vi "OCT Bscan Test_2.vi"() -> ()   [LabVIEW 2017]
panel:
  out "Intensity Graph":dbl[][](graph)
  in  "Data Range":T1={"Z start (pxl)"=1, "Z length (pxl)"=400}
  in  "# Cscan":i32
  in  "Save Path":path=path "E:/Jiarui/0212test"
  out "error out":errorcluster
  in  "Objective":u16(ring)=1 items=["5X LKM05", "10X LKM10", "20X LKM20", "10X LSM02"]
  in  "ROI Parameters":T2={"ROI (mm)"={"X (mm)"=1.0, "Y (mm)"=1.0}, "Shift (mm)"={"Xshift (mm)"=0.0, "Yshift (mm)"=0.0}}
  in  "Scan Parameters":T3={"# Scan"={"#Ascan"=400, "#Bscan"=400}, "# Rpt"={"#ARpt"=1, "#BRpt"=1}, "Aline Rate"=2, "# Extra"={"# ARpt_extra"=5, "#Brtn_extra"=80}} {"Aline Rate" items=["76 KHz", "146 KHz", "76 KHz", "28 KHz", "10 KHz"]}
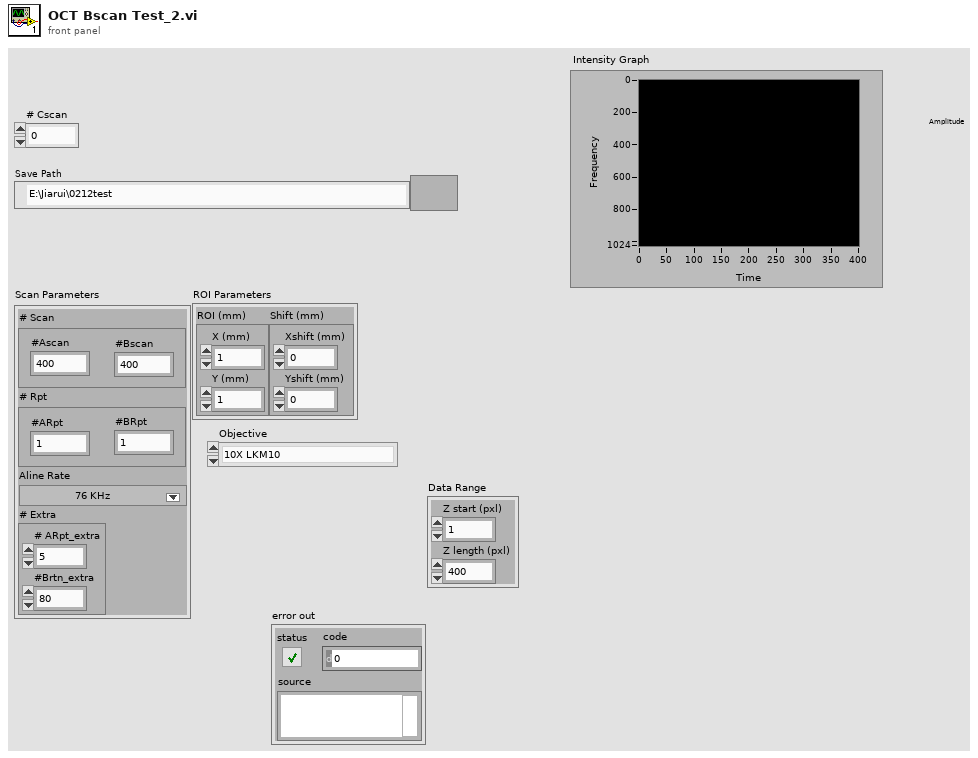
[diagram p1: front panel]
types:
  T1 = cluster{"Z start (pxl)":i32, "Z length (pxl)":i32}
  T2 = cluster{"ROI (mm)":cluster{"X (mm)":sgl, "Y (mm)":sgl}, "Shift (mm)":cluster{"Xshift (mm)":sgl, "Yshift (mm)":sgl}}
  T3 = cluster{"# Scan":cluster{"#Ascan":i32, "#Bscan":i32}, "# Rpt":cluster{"#ARpt":i32, "#BRpt":i32}, "Aline Rate":u16, "# Extra":cluster{"# ARpt_extra":i32, "#Brtn_extra":i32}}
  T4 = enum16{"Init", "Configure", "Configure Data", "Generate Scan Pattern", "Start Acquire Raw", "Start Acquire Data", "Acquire RAW", "Acquire Data", "Stop Acquire", "Uninit"}
  T5 = enum16{"Create", "Enqueue", "Dequeue", "Release"}
  T6 = cluster{"Image Index":i16, "Slice Index":i16, "#Cscan":i32, "nAT per B":i32, "nA per B":i32, "Brtn_extra/2":i32}
  T7 = cluster{"Objective":u16, "Aline Rate":u16, "# Cscan":i32, "ROI Parameters":cluster{"ROI (mm)":cluster{"X (mm)":sgl, "Y (mm)":sgl}, "Shift (mm)":cluster{"Xshift (mm)":sgl, "Yshift (mm)":sgl}}}
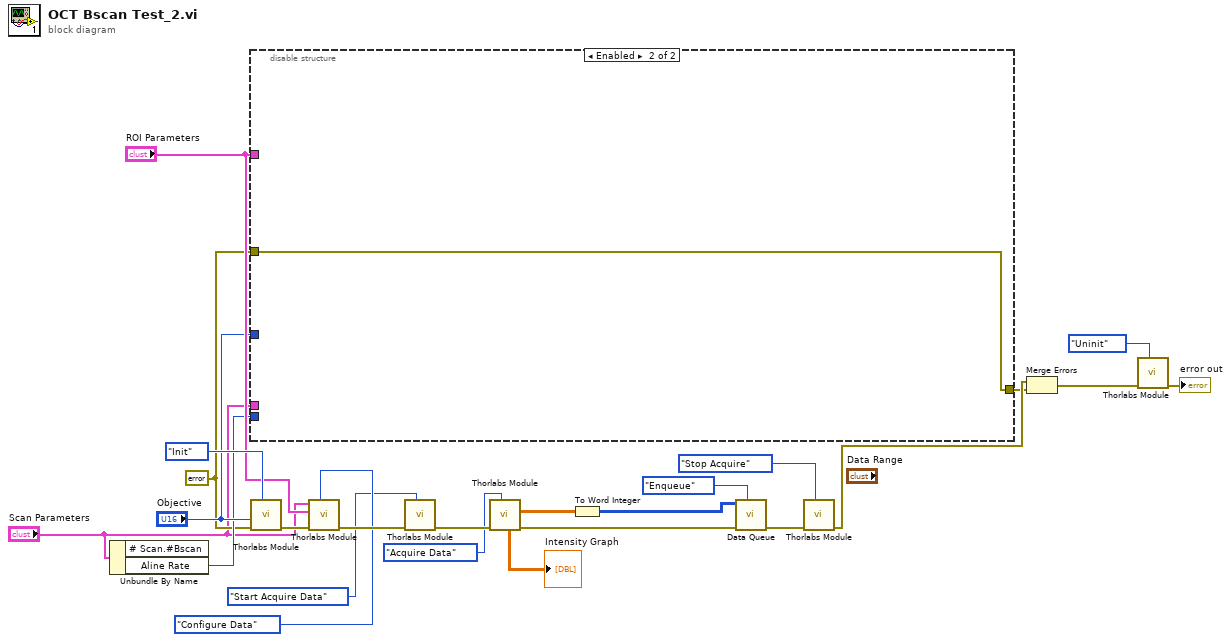
[diagram p0: block diagram]
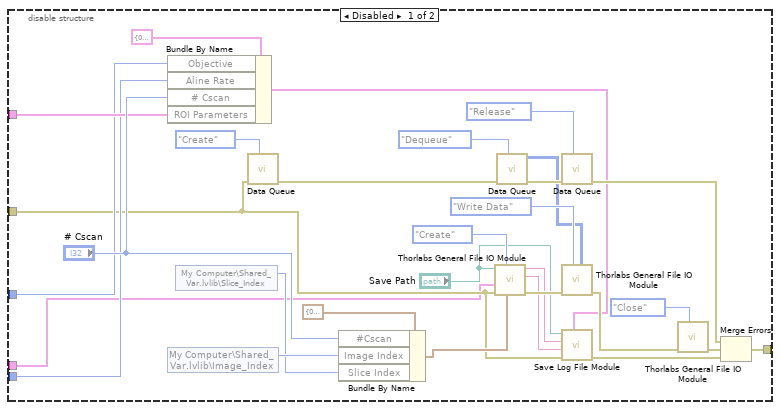
[diagram p2: hidden frame]
diagram:
  w6 = errorcluster {"status"=FALSE, "code"=0, "source"=""} ("error in")
  n1 = Unbundle By Name("Scan Parameters") -> ("Aline Rate"=w11:u16)  [unwired: 1 out]
  n2 = disable-structure shown="Enabled" {
    disable-tunnel: "ROI Parameters" -> [w33 _]
    disable-tunnel: "Objective" -> [w32 _]
    disable-tunnel: w11 -> [w31 _]
    disable-tunnel: [w30 w55] -> w7
    disable-tunnel: w6 -> [w27 w55]
    disable-tunnel: "Scan Parameters" -> [w26 _]
    frame Disabled {
      n3 = Bundle By Name(cluster=T7 {"Objective"=0, "Aline Rate"=2, "# Cscan"=1, "ROI Parameters"={"ROI (mm)"={"X (mm)"=1.0, "Y (mm)"=1.0}, "Shift (mm)"={"Xshift (mm)"=0.0, "Yshift (mm)"=0.0}}} ("Log Header Parameters"), "Objective"=w32, "Aline Rate"=w31, "# Cscan"="# Cscan", "ROI Parameters"=w33) -> (w45:T7)
      n4 = shared-variable "My Computer\\Shared_Var.lvlib\\Image_Index"() -> (w40:i16)  [unwired: 1 in, 1 out]
      n5 = shared-variable "My Computer\\Shared_Var.lvlib\\Slice_Index"() -> (w39:i16)  [unwired: 1 in, 1 out]
      n6 = call "Data Queue.vi"("Action"=T5."Create", "error in (no error)"=w27) -> ("error out"=w50:errorcluster)  [unwired: 8 in, 1 out]
      n7 = Bundle By Name(cluster=T6 {"Image Index"=0, "Slice Index"=0, "#Cscan"=0, "nAT per B"=0, "nA per B"=0, "Brtn_extra/2"=0} ("Imaging Parameters"), "#Cscan"="# Cscan", "Image Index"=w40, "Slice Index"=w39) -> (w38:T6)
      n8 = call "Thorlabs General File IO Module.vi"("Imaging Parameters"=w38, "Actions"=enum16{"Create", "Write", "Write Data", "Close"}."Create", "error in"=w27, "Scan Parameters"=w26, "Save Path"="Save Path") -> ("error out"=w49:errorcluster, "Scan Parameter"=w43:string, "Save Name"=w44:string)  [unwired: 4 in]
      n9 = call "Data Queue.vi"("Action"=T5."Dequeue", "error in (no error)"=w50) -> ("error out"=w52:errorcluster, "Data Out"=w25:i16[][])  [unwired: 8 in]
      n10 = call "Data Queue.vi"("Action"=T5."Release", "error in (no error)"=w52) -> ("error out"=w54:errorcluster)  [unwired: 8 in, 1 out]
      n11 = call "Thorlabs General File IO Module.vi"("Data In"=w25, "Actions"=enum16{"Create", "Write", "Write Data", "Close"}."Write Data", "error in"=w49) -> ("error out"=w48:errorcluster)  [unwired: 6 in, 2 out]
      n12 = call "Save Log File Module.vi"("Log Header Parameters"=w45, "error in (no error)"=w27, "Scan Parameter"=w43, "Save Name"=w44, "Save Path"="Save Path") -> ("error out"=w42:errorcluster)  [unwired: 6 in]
      n13 = call "Thorlabs General File IO Module.vi"("Actions"=enum16{"Create", "Write", "Write Data", "Close"}."Close", "error in"=w48) -> ("error out"=w47:errorcluster)  [unwired: 7 in, 2 out]
      n14 = Merge Errors(w54, w47, w42) -> (w30:errorcluster)
    }
    frame Enabled {
    }
  }
  n15 = call "Thorlabs Module.vi"("Actions"=T4."Init", "error in"=w6, "Objective"="Objective") -> ("error out"=w24:errorcluster)  [unwired: 5 in, 3 out]
  n16 = call "Thorlabs Module.vi"("Actions"=T4."Configure Data", "error in"=w24, "ROI Parameters"="ROI Parameters", "Scan Parameters"="Scan Parameters") -> ("error out"=w23:errorcluster)  [unwired: 4 in, 3 out]
  n17 = call "Thorlabs Module.vi"("Actions"=T4."Start Acquire Data", "error in"=w23) -> ("error out"=w22:errorcluster)  [unwired: 6 in, 3 out]
  n18 = call "Thorlabs Module.vi"("Actions"=T4."Acquire Data", "error in"=w22) -> ("error out"=w10:errorcluster, "Data Out"=w2:sgl[][], "Intensity Graph"=→"Intensity Graph":dbl[][])  [unwired: 6 in, 1 out]
  n19 = To Word Integer(number=w2) -> (16bit integer=w3:i16[][])
  n20 = call "Data Queue.vi"("Action"=T5."Enqueue", "error in (no error)"=w10, "Data In"=w3) -> ("error out"=w18:errorcluster)  [unwired: 7 in, 1 out]
  n21 = call "Thorlabs Module.vi"("Actions"=T4."Stop Acquire", "error in"=w18) -> ("error out"=w21:errorcluster)  [unwired: 6 in, 3 out]
  n22 = Merge Errors(w21, w7) -> (w20:errorcluster)
  n23 = call "Thorlabs Module.vi"("Actions"=T4."Uninit", "error in"=w20) -> ("error out"=→"error out":errorcluster)  [unwired: 6 in, 3 out]
